vi "Get Power Regulation.vi"(2 "shared":refnum<class "niUSRP Rx Core v1 FPGA.lvclass">=refnum) -> (4 "power regulation":refnum<class "niVST Power Regulation v1 FPGA.lvclass">)   [LabVIEW 2023]
uses:
  <instrlib>/niVST/Power Regulation/Interface/v1/FPGA/niVST Power Regulation v1 FPGA.lvclass
  <instrlib>/niUSRP/Reference FPGA/Rx Core/niUSRP Rx Core v1 FPGA.lvclass
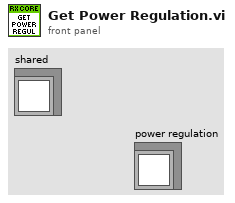
[diagram p1: front panel]
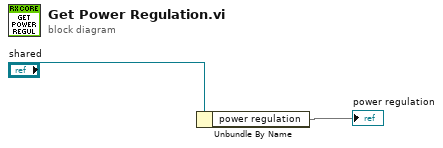
[diagram p0: block diagram]
diagram:
  n1 = Unbundle By Name("shared") -> ("power regulation"=→"power regulation")
